vi "_backward add grad.vi"(7 "In":refnum<class "Value.lvclass">, 8 "error in":errorcluster, 10 "out grad":T1, 11 "variant":variant) -> (0 "error out":errorcluster, 3 "out":variant)   [LabVIEW 2023, in "LabGRAD.lvlib" / "Value.lvclass"]
uses:
  Value.lvclass
  Value.lvclass/Value.ctl
  UiObjects/numeric value control.ctl
  UiObjects/UiObjects.lvclass
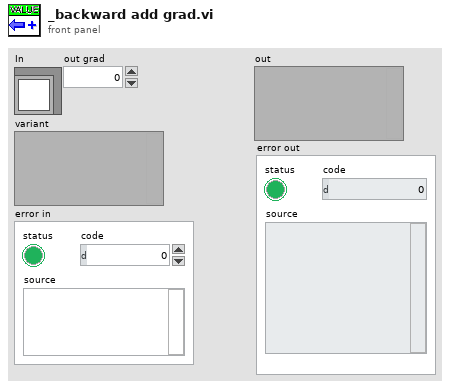
[diagram p1: front panel]
types:
  T1 = typedef "UiObjects.lvlib/UiObjects.lvclass/numeric value control.ctl" = dbl
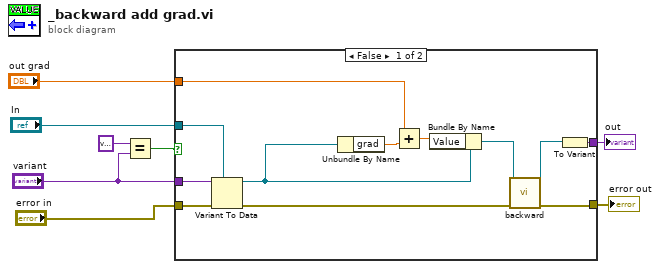
[diagram p0: block diagram]
diagram:
  n1 = Equal?(x=variant, y="variant") -> (x = y?=w1:bool)
  n2 = case shown="False" w1 {
    tunnel: "variant" -> [w19 w21]
    tunnel: "In" -> [w18 _]
    tunnel: "out grad" -> [w16 _]
    tunnel: [w14 w21] -> w6
    tunnel: "error in" -> [w13 w22]
    tunnel: [w11 w22] -> w4
    frame False {
      n3 = Variant To Data(error in=w13, type=w18, Variant=w19) -> (data=w15:refnum<class "Value.lvclass">, error out=w12:errorcluster)
      n4 = Unbundle By Name(w15) -> ("grad"=w17:T1)
      n5 = Add(x=w16, y=w17) -> (x+y=w20:T1)
      n6 = Bundle By Name(cluster=w15, "Value"=w20) -> (w10:refnum<class "Value.lvclass">)
      n7 = call "backward.vi"("i"=w12, "In"=w10) -> ("error out"=w11:errorcluster, "Out"=w9:refnum<class "Value.lvclass">)  [unwired: 8 in]
      n8 = To Variant(anything=w9) -> (Variant=w14:variant)
    }
    frame True {
      # "this vi needs protection from casting an \nempty var"
    }
  }
  "out" <- w6
  "error out" <- w4
